vi "Enum.vi"() -> ()   [LabVIEW 2019]
panel:
  in  "Enum 2":T1(ring)
  out "EnumIndicator":u8
  in  "Enum":enum16{"Jan", "Feb", "Mar", "Apr", "May"}(ring)
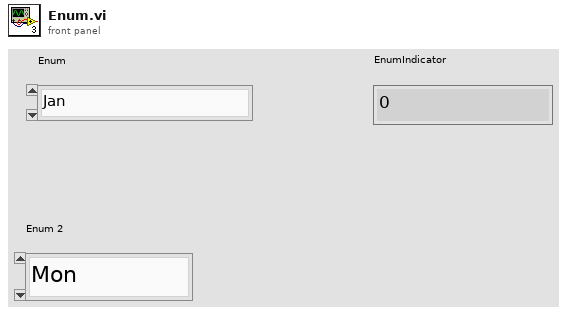
[diagram p1: front panel]
types:
  T1 = enum16{"Mon", "Tue", "Wed", "Thu", "Fri", "Sat", "Sun"}
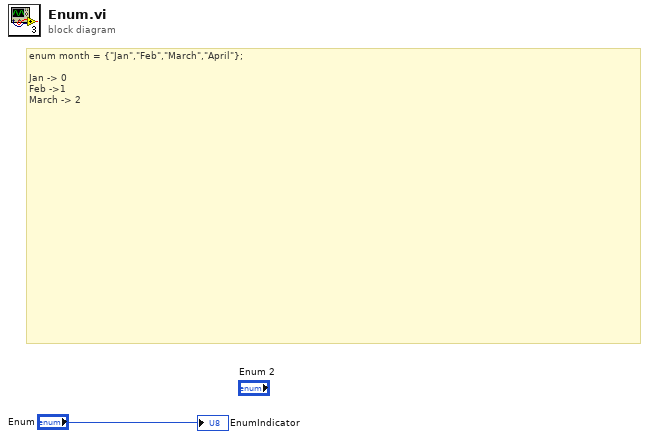
[diagram p0: block diagram]
diagram:
  # "enum month = {\"Jan\",\"Feb\",\"March\",\"April\"};\n\nJan -> 0\nFeb ->1\nMarch -> 2"
  "EnumIndicator" <- "Enum"
